vi "Add Files to Archive.vi"(8 "error in (no error)":errorcluster, 9 "relative paths in zip":path[](array[path]), 10 "absolute source paths":path[](array[path]), 11 "zip path":path) -> (0 "error out":errorcluster)   [LabVIEW 2021]
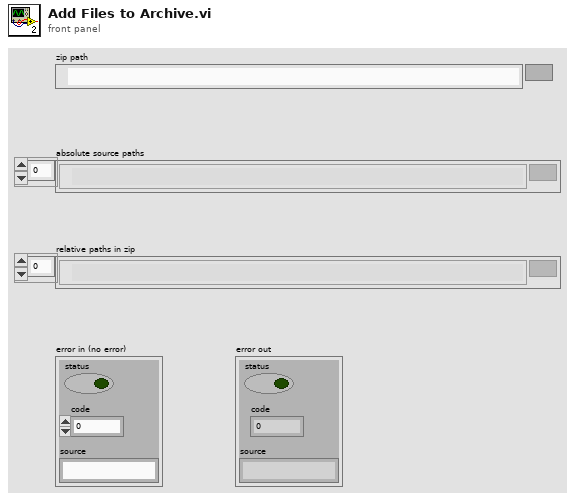
[diagram p1: front panel]
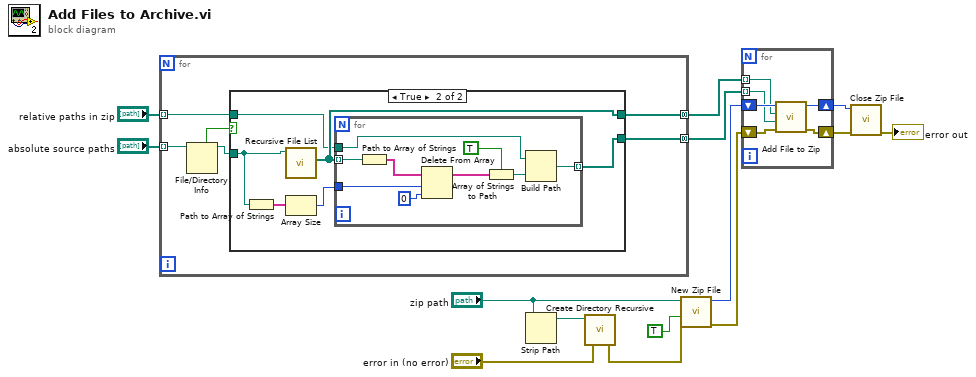
[diagram p0: block diagram]
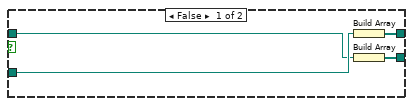
[diagram p2: hidden frame]
diagram:
  n1 = for {
    tunnel: [w18] -> w6 mode=concatenating
    tunnel: "absolute source paths" -> [w17] mode=indexing
    tunnel: "relative paths in zip" -> [w16] mode=indexing
    tunnel: [w15] -> w5 mode=concatenating
    n2 = File/Directory Info(path=w17) -> (path out=w19:path, directory=w20:bool)  [unwired: 1 in, 5 out]
    n3 = case shown="True" w20 {
      tunnel: w19 -> [w24 w26]
      tunnel: [w23 w30] -> w18
      tunnel: w16 -> [w22 w25]
      tunnel: [w21 w29] -> w15
      frame False {
        n4 = Build Array(w24) -> (w23:path[])
        n5 = Build Array(w22) -> (w21:path[])
      }
      frame True {
        n6 = Path to Array of Strings(0:w26) -> (2:w28:string[])  [unwired: 1 out]
        n7 = call <vilib>:"Recursive File List.vi"("Folder Path"=w26) -> ("All Files in Dir"=w30:path[])  [unwired: 6 in, 4 out]
        n8 = Array Size(array=w28) -> (size(s)=w27:i32)
        n9 = for {
          tunnel: w30 -> [w39] mode=indexing
          tunnel: [w37] -> w29 mode=indexing
          tunnel: w27 -> [w38]
          tunnel: w25 -> [w31]
          n10 = Path to Array of Strings(0:w39) -> (2:w35:string[])  [unwired: 1 out]
          n11 = Delete From Array(array=w35, length=w38, index=0 ("length")) -> (array with subset deleted=w33:string[])  [unwired: 1 out]
          n12 = Array of Strings to Path(0:w33, 1:TRUE ("relative")) -> (2:w32:path)
          n13 = Build Path(base path=w31, name or relative path=w32) -> (appended path=w37:path)
        }
      }
    }
  }
  n14 = Strip Path(path="zip path") -> (stripped path=w3:path)  [unwired: 1 out]
  n15 = call <vilib>:"Create Directory Recursive.vi"("error in (no error)"="error in (no error)", "directory"=w3) -> ("error out"=w1:errorcluster)  [unwired: 3 in, 2 out]
  n16 = call <vilib>:"New Zip File.vi"("error in (no error)"=w1, "confirm overwrite? (F)"=TRUE, "target"="zip path") -> ("error out"=w13:errorcluster, "zip file out"=w9:i64)  [unwired: 2 in, 1 out]
  n17 = for {
    tunnel: w6 -> [w40] mode=indexing
    shift-right: [w41] -> w12
    shift-left: w13 -> [w43]
    shift-right: [w44] -> w11
    shift-left: w9 -> [w45]
    tunnel: w5 -> [w42] mode=indexing
    n18 = call <vilib>:"Add File to Zip.vi"("error in (no error)"=w43, "destination path in zip"=w42, "source file path"=w40, "zip file in"=w45) -> ("error out"=w41:errorcluster, "zip file out"=w44:i64)  [unwired: 6 in]
  }
  n19 = call <vilib>:"Close Zip File.vi"("error in (no error)"=w12, "zip file in"=w11) -> ("error out"=→"error out":errorcluster)  [unwired: 5 in]
